vi "TCP Data Client.vi"() -> ()   [LabVIEW 2010]
doc: "Displays data sent via TCP from Data Server.vi. Once a TCP connection is open, the VI reads 4 bytes to determine the amount of data being sent. It then reads and charts that many bytes. If an error occurs or the stop button is pressed, it sends a \"Q\" to the Data Sender to notify it to quit.\n\n<B>Note:</B> Requires the Data Server.vi located in the same library as this VI."
uses:
  5.0-Global.vi
panel:
  out "XY Graph":cluster{sgl[], sgl[]}(graph)
  in  "Address":string="10.10.10.2"
  in  "Port":u16=33483 min=1025 step=1
  # "Instructions:\n1. Open the Data Server.vi located in the same library.\n2. Follow the instructions on it's front panel.\n\nNote: This VI is built to work with the Data Server.vi."
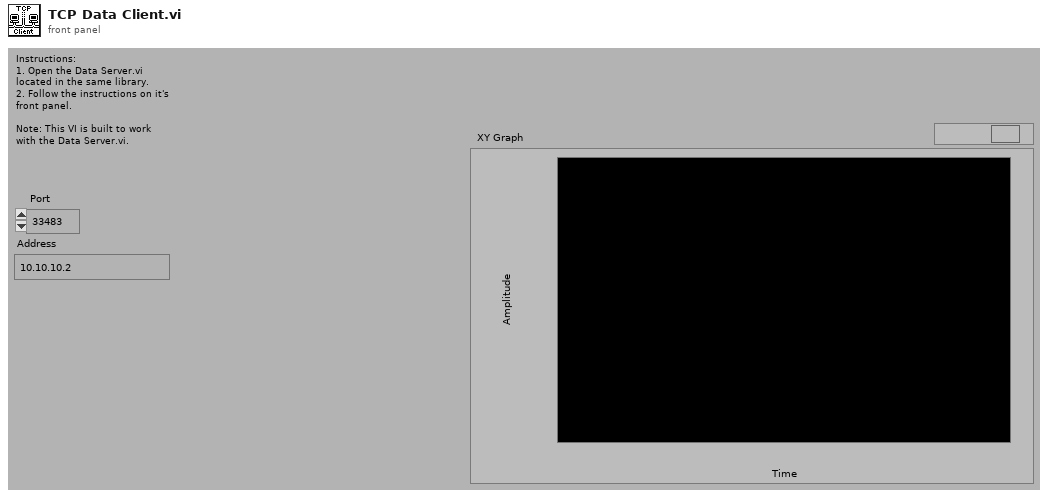
[diagram p1: front panel]
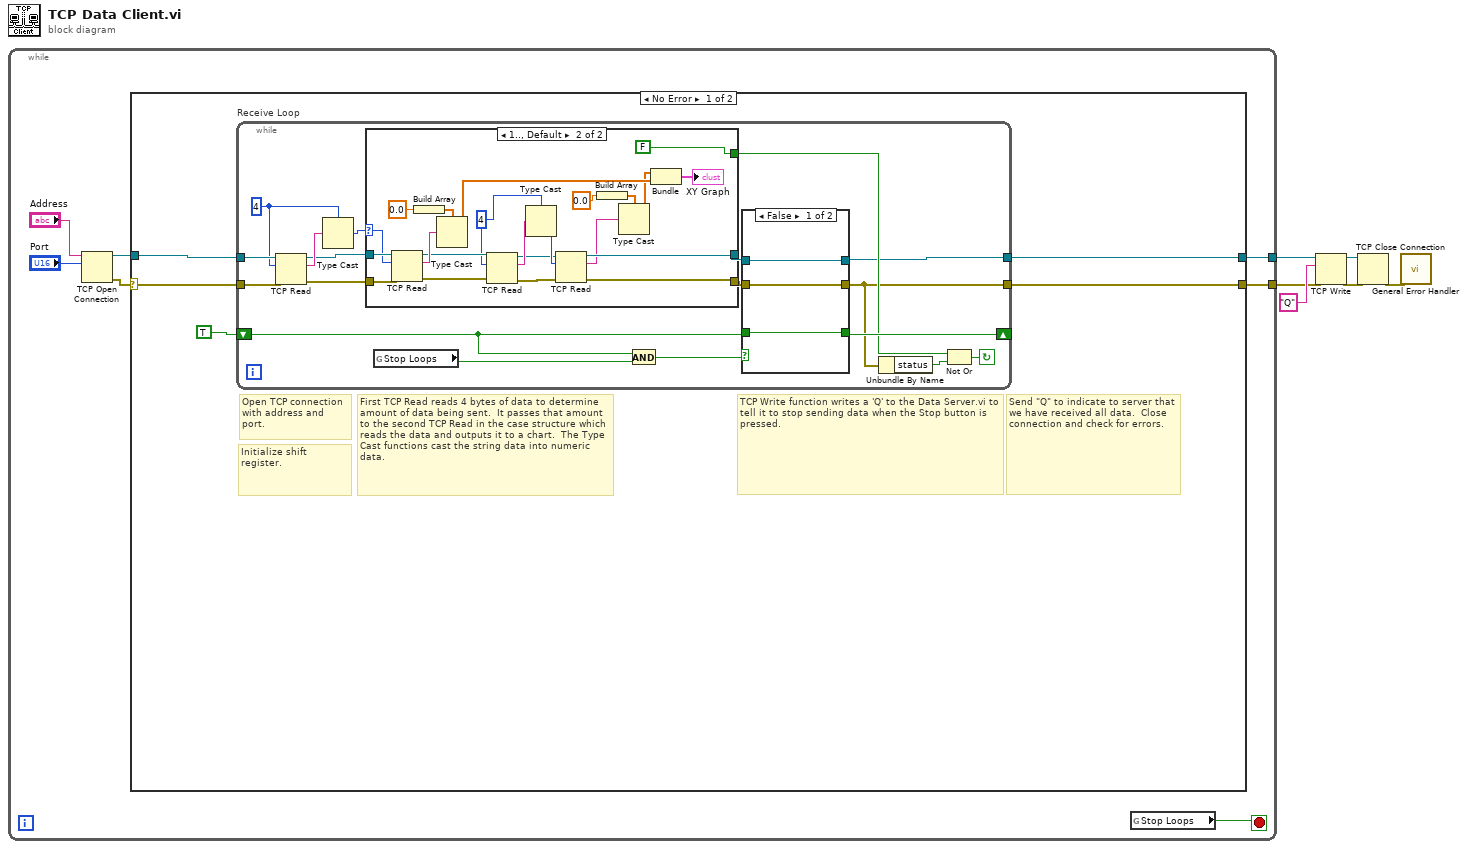
[diagram p0: block diagram]
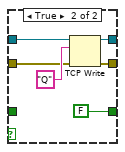
[diagram p2: hidden frame]
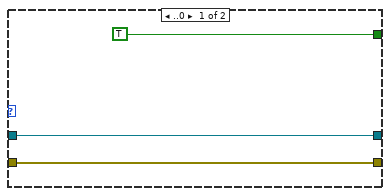
[diagram p3: hidden frame]
diagram:
  n1 = while {
    tunnel: [w9] -> w2
    tunnel: [w8] -> w1
    stop <- w7 stop-if-true
    n2 = TCP Open Connection(address="Address", remote port or service name="Port") -> (connection ID=w11:refnum<k5>, error out=w10:errorcluster)  [unwired: 1 in, 2 out]
    n3 = case shown="No Error" w10 {
      selector: w10 -> [w17 w71]
      tunnel: w11 -> [w14 w72]
      tunnel: [w16 w72] -> w9
      tunnel: [w15 w71] -> w8
      frame No Error {
        # "Send \"Q\" to indicate to server that we have received all data.  Close connection and check for errors."
        # "TCP Write function writes a 'Q' to the Data Server.vi to tell it to stop sending data when the Stop button is pressed."
        # "First TCP Read reads 4 bytes of data to determine amount of data being sent.  It passes that amount to the second TCP Read in the case structure which reads the data and outputs it to a chart.  The Type Cast functions cast the string data into numeric data."
        # "Initialize shift register."
        # "Open TCP connection with address and port."
        n4 = while "Receive Loop" {
          shift-left: TRUE -> [w22]
          shift-right: [w29] -> _
          tunnel: w17 -> [w33]
          tunnel: w14 -> [w34]
          tunnel: [w24] -> w16
          tunnel: [w21] -> w15
          stop <- w35 continue-if-true
          w32 = 4
          n5 = TCP Read(connection ID=w34, bytes to read=w32, error in (no error)=w33) -> (connection ID out=w25:refnum<k5>, data out=w36:string, error out=w26:errorcluster)  [unwired: 2 out]
          n6 = Type Cast(type=w32, x=w36) -> (*(type *) &x=w31:i32)
          n7 = case shown="1.., Default" w31 {
            selector: w31 -> [_ w67]
            tunnel: w26 -> [w46 w69]
            tunnel: w25 -> [w48 w68]
            tunnel: [w48 w60] -> w23
            tunnel: [TRUE FALSE] -> w27
            tunnel: [w46 w61] -> w28
            frame ..0 {
            }
            frame 1.., Default {
              w58 = 4
              n8 = TCP Read(connection ID=w68, bytes to read=w67, error in (no error)=w69) -> (connection ID out=w63:refnum<k5>, data out=w70:string, error out=w62:errorcluster)  [unwired: 2 out]
              n9 = Build Array(sgl 0.0) -> (w64:sgl[])
              n10 = Type Cast(type=w64, x=w70) -> (*(type *) &x=w51:sgl[])
              n11 = TCP Read(connection ID=w63, bytes to read=w58, error in (no error)=w62) -> (connection ID out=w55:refnum<k5>, data out=w59:string, error out=w56:errorcluster)  [unwired: 2 out]
              n12 = Type Cast(type=w58, x=w59) -> (*(type *) &x=w57:i32)
              n13 = TCP Read(connection ID=w55, bytes to read=w57, error in (no error)=w56) -> (connection ID out=w60:refnum<k5>, data out=w52:string, error out=w61:errorcluster)  [unwired: 2 out]
              n14 = Build Array(sgl 0.0) -> (w54:sgl[])
              n15 = Type Cast(type=w54, x=w52) -> (*(type *) &x=w50:sgl[])
              n16 = Bundle(w50, w51) -> (→"XY Graph":cluster{sgl[], sgl[]})  [unwired: 1 in]
            }
          }
          n17 = global read "5.0-Global.vi" "Stop Loops"() -> (w19:bool)
          n18 = And(x=w22, y=w19) -> (x .and. y?=w30:bool)
          n19 = case shown="False" w30 {
            tunnel: w22 -> [w38 _]
            tunnel: [w38 FALSE] -> w29
            tunnel: w23 -> [w37 w45]
            tunnel: w28 -> [w39 w42]
            tunnel: [w39 w41] -> w21
            tunnel: [w37 w40] -> w24
            frame False {
            }
            frame True {
              n20 = TCP Write(connection ID=w45, data in="Q", error in (no error)=w42) -> (connection ID out=w40:refnum<k5>, error out=w41:errorcluster)  [unwired: 2 out]
            }
          }
          n21 = Unbundle By Name(w21) -> ("status"=w20:bool)
          n22 = Not Or(1:w20, 2:w27) -> (0:w35:bool)
        }
      }
      frame Error {
      }
    }
    n23 = global read "5.0-Global.vi" "Stop Loops"() -> (w7:bool)
  }
  n24 = TCP Write(connection ID=w2, data in="Q", error in (no error)=w1) -> (connection ID out=w6:refnum<k5>, error out=w5:errorcluster)  [unwired: 2 out]
  n25 = TCP Close Connection(connection ID=w6, error in (no error)=w5) -> (error out=w3:errorcluster)  [unwired: 2 out]
  n26 = call <vilib>:"General Error Handler.vi"("error in (no error)"=w3) -> ()  [unwired: 1 in, 14 out]
